vi "Init Sessions.vi"(8 "error in (no error)":errorcluster, 11 "Server in":refnum<class "Server.lvclass">) -> (0 "error out":errorcluster, 3 "Server out":refnum<class "Server.lvclass">)   [LabVIEW 2020, in "HTTP Server.lvlib" / "Server.lvclass"]
uses:
  Server.lvclass
  Request Session Handler/Request Session Handler.lvclass
  C:/dev/IlluminatedG/lv-http-server/HTTP Server/Handler/Handler.lvclass
  Session Cleanup Handler/Session Cleanup Handler.lvclass
  Session Response Handler/Session Response Handler.lvclass
  Add Connection Handler.vi
  Add Request Handler.vi
  Add Route Handler.vi
  Add Controller Handler.vi
  Add Controller.vi
  Add Response Handler.vi
  Add Complete Handler.vi
  Add Exception Handler.vi
  Connection Handler/Connection Handler.lvclass
  Request Handler/Request Handler.lvclass
  Route Handler/Route Handler.lvclass
  Controller Handler/Controller Handler.lvclass
  Controller/Controller.lvclass
  Response Handler/Response Handler.lvclass
  Complete Handler/Complete Handler.lvclass
  Exception Handler/Exception Handler.lvclass
  Handler/Handler.lvclass
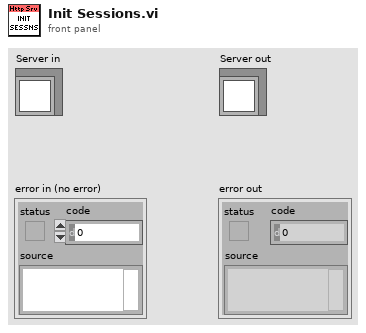
[diagram p1: front panel]
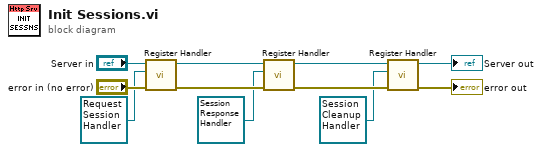
[diagram p0: block diagram]
diagram:
  n1 = call "Register Handler.vi"("error in (no error)"="error in (no error)", "Handler"=refnum<class "Request Session Handler.lvclass"> refnum ("HTTP Server.lvlib:Request Session Handler.lvclass"), "Server in"="Server in") -> ("error out"=w7:errorcluster, "Server out"=w8:refnum<class "Server.lvclass">)  [unwired: 7 in]
  n2 = call "Register Handler.vi"("error in (no error)"=w7, "Handler"=refnum<class "Session Response Handler.lvclass"> refnum ("HTTP Server.lvlib:Session Response Handler.lvclass"), "Server in"=w8) -> ("error out"=w6:errorcluster, "Server out"=w4:refnum<class "Server.lvclass">)  [unwired: 7 in]
  n3 = call "Register Handler.vi"("error in (no error)"=w6, "Handler"=refnum<class "Session Cleanup Handler.lvclass"> refnum ("HTTP Server.lvlib:Session Cleanup Handler.lvclass"), "Server in"=w4) -> ("error out"=→"error out":errorcluster, "Server out"=→"Server out":refnum<class "Server.lvclass">)  [unwired: 7 in]
